vi "pmu_Build Time Quality Flag.vi"(0 "unlocked seconds":u32, 1 "synchronization error (s)":dbl=1e-07 format="%#_15f", 5 "locked?":bool, 7 "leap second pending":bool, 9 "leap second occurred":bool, 11 "leap second direction":bool) -> (4 "time quality flag":u8 format="%08b", 6 "PMU time quality":u8 format="%08b")   [LabVIEW 2013, in "NI_EP_PMU.lvlib"]
doc: "Outputs time quality flag bits, according to IEEE Std C37.118."
uses:
  <vilib>/addons/Electrical Power/PMU/NI_EP_PMU.lvlib
panel:
  # "100 ns"
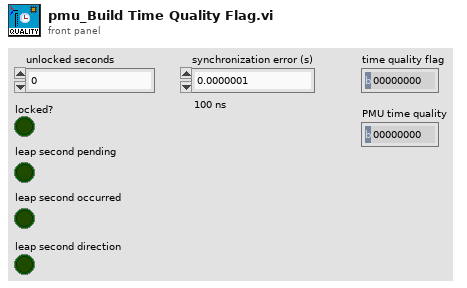
[diagram p1: front panel]
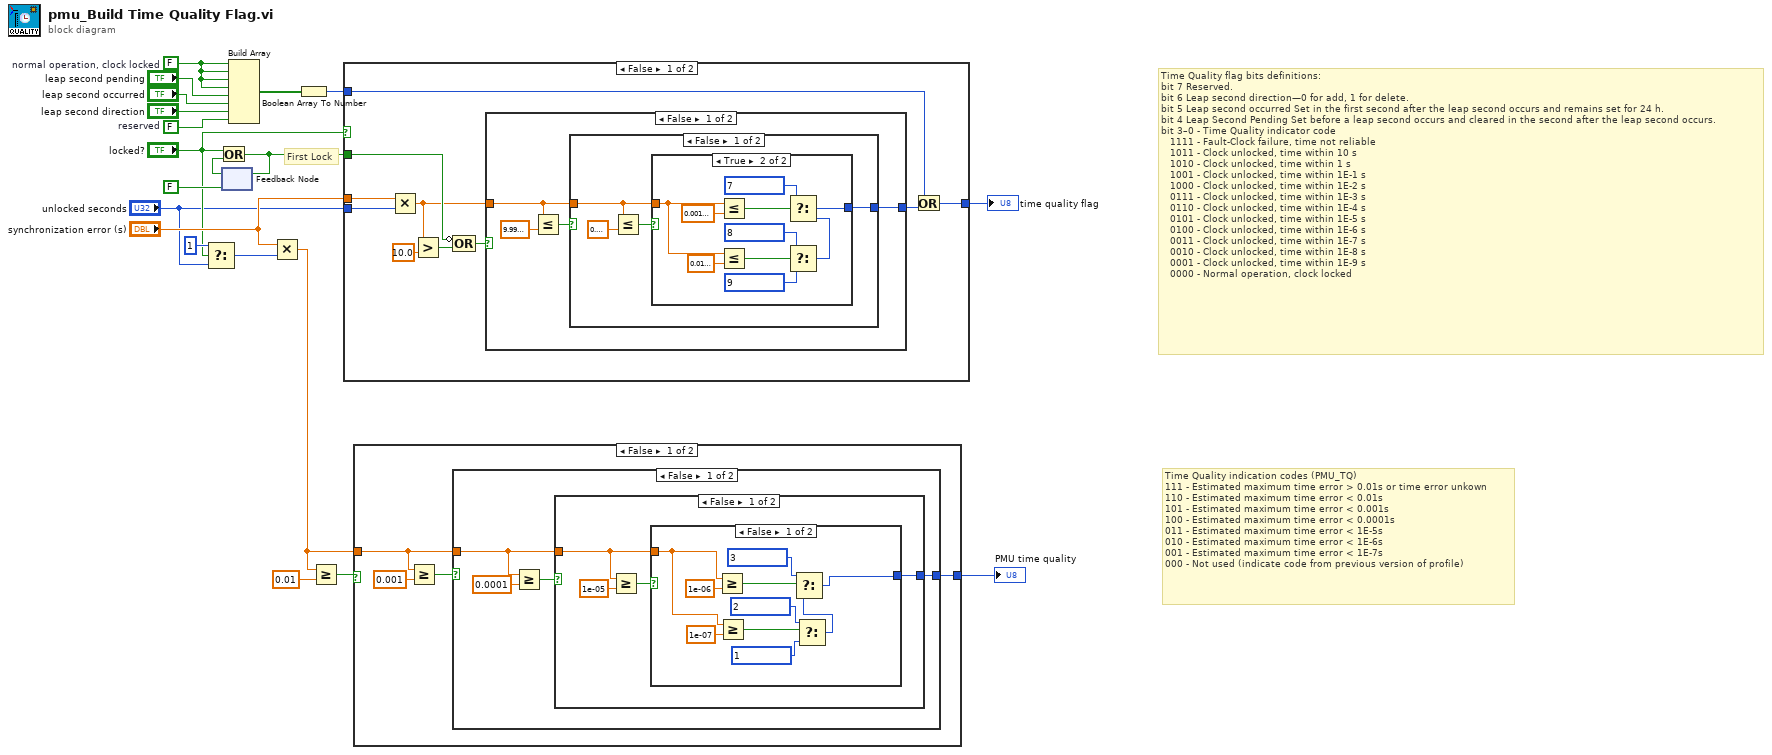
[diagram p0: block diagram]
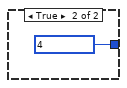
[diagram p2: hidden frame]
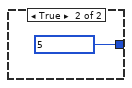
[diagram p3: hidden frame]
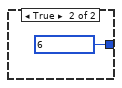
[diagram p4: hidden frame]
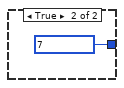
[diagram p5: hidden frame]
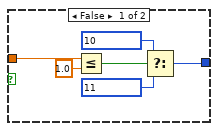
[diagram p6: hidden frame]
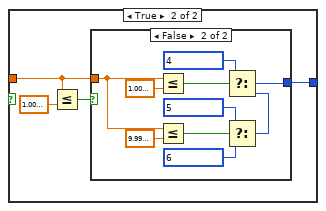
[diagram p7: hidden frame]
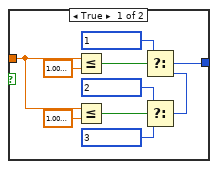
[diagram p8: hidden frame]
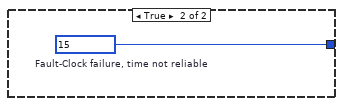
[diagram p9: hidden frame]
diagram:
  w11 = FALSE  # normal operation, clock locked
  w10 = FALSE  # reserved
  # "Time Quality indication codes (PMU_TQ)\n111 - Estimated maximum time error > 0.01s or time error unkown\n110 - Estimated maximum time error < 0.01s\n101 - Estimated maximum time error < 0.001s\n100 - Estimated maximum time error < 0.0001s\n011 - Estimated maximum time error < 1E-5s\n010 - Estimated maximum time error < 1E-6s\n001 - Estimated maximum time error < 1E-7s\n000 - Not used (indicate code from previous version of profile)"
  # "First Lock"
  # "Time Quality flag bits definitions:\nbit 7 Reserved.\nbit 6 Leap second direction—0 for add, 1 for delete.\nbit 5 Leap second occurred Set in the first second after the leap second occurs and remains set for 24 h.\nbit 4 Leap Second Pending Set before a leap second occurs and cleared in the second after the leap second occurs.\nbit 3–0 - Time Quality indicator code\n   1111 - Fault-Clock failure, time not reliable\n   1011 - Clock unlocked, time within 10 s\n   1010 - Clock unlocked, time within 1 s\n   1001 - Clock unlocked, time within 1E-1 s\n   1000 - Clock unlocked, time within 1E-2 s\n   0111 - Clock unlocked, time within 1E-3 s\n   0110 - Clock unlocked, time within 1E-4 s\n   0101 - Clock unlocked, time within 1E-5 s\n   0100 - Clock unlocked, time within 1E-6 s\n   0011 - Clock unlocked, time within 1E-7 s\n   0010 - Clock unlocked, time within 1E-8 s\n   0001 - Clock unlocked, time within 1E-9 s\n   0000 - Normal operation, clock locked"
  n1 = Select(t=u32 1, s="locked?", f="unlocked seconds") -> (s? t:f=w1:u32)
  n2 = feedback #1(FALSE) -> (w19:bool)
  n3 = Or(x="locked?", y=w19) -> (x .or. y?=w16:bool)
  n4 = feedback-in #1(w16) -> ()
  n5 = Build Array(w11, w11, w11, w11, "leap second pending", "leap second occurred", "leap second direction", w10) -> (w18:bool[])
  n6 = Multiply(x="synchronization error (s)", y=w1) -> (x*y=w5:dbl)
  n7 = Boolean Array To Number(Boolean array=w18) -> (number=w17:u8)
  n8 = Greater Or Equal?(x=w5, y=0.01) -> (x >= y?=w8:bool)
  n9 = case shown="False" "locked?" {
    tunnel: "unlocked seconds" -> [w22 _]
    tunnel: [w24 w80] -> w15
    tunnel: w17 -> [w25 w80]
    tunnel: w16 -> [w28 _]
    tunnel: "synchronization error (s)" -> [w21 _]
    frame False {
      n10 = Multiply(x=w21, y=w22) -> (x*y=w27:dbl)
      n11 = Greater?(x=w27, y=10.0) -> (0:w29:bool)
      n12 = Compound Arithmetic op=OR(invert w28, w29) -> (w26:bool)
      n13 = case shown="False" w26 {
        tunnel: [w31 w79] -> w23
        tunnel: w27 -> [w32 _]
        frame False {
          n14 = Less Or Equal?(x=w32, y=9.999999999976694e-05) -> (x <= y?=w33:bool)
          n15 = case shown="False" w33 {
            tunnel: w32 -> [w36 w56]
            tunnel: [w35 w55] -> w31
            frame False {
              n16 = Less Or Equal?(x=w36, y=0.10000000000000142) -> (x <= y?=w37:bool)
              n17 = case shown="True" w37 {
                tunnel: w36 -> [w43 w49]
                tunnel: [w39 w51] -> w35
                frame False {
                  n18 = Less Or Equal?(x=w43, y=1.0) -> (x <= y?=w42:bool)
                  n19 = Select(t=u8 10, s=w42, f=u8 11) -> (s? t:f=w39:u8)
                }
                frame True {
                  n20 = Less Or Equal?(x=w49, y=0.0010000000000012221) -> (x <= y?=w53:bool)
                  n21 = Less Or Equal?(x=w49, y=0.010000000000001563) -> (x <= y?=w48:bool)
                  n22 = Select(t=u8 8, s=w48, f=u8 9) -> (s? t:f=w45:u8)
                  n23 = Select(t=u8 7, s=w53, f=w45) -> (s? t:f=w51:u8)
                }
              }
            }
            frame True {
              n24 = Less Or Equal?(x=w56, y=1.0000000116860974e-07) -> (x <= y?=w57:bool)
              n25 = case shown="False" w57 {
                tunnel: w56 -> [w63 w73]
                tunnel: [w65 w75] -> w55
                frame True {
                  n26 = Less Or Equal?(x=w63, y=1.000000082740371e-09) -> (x <= y?=w67:bool)
                  n27 = Less Or Equal?(x=w63, y=1.000000082740371e-08) -> (x <= y?=w62:bool)
                  n28 = Select(t=u8 2, s=w62, f=u8 3) -> (s? t:f=w59:u8)
                  n29 = Select(t=u8 1, s=w67, f=w59) -> (s? t:f=w65:u8)
                }
                frame False {
                  n30 = Less Or Equal?(x=w73, y=1.0000000010279564e-06) -> (x <= y?=w77:bool)
                  n31 = Less Or Equal?(x=w73, y=9.999999999621423e-06) -> (x <= y?=w72:bool)
                  n32 = Select(t=u8 5, s=w72, f=u8 6) -> (s? t:f=w69:u8)
                  n33 = Select(t=u8 4, s=w77, f=w69) -> (s? t:f=w75:u8)
                }
              }
            }
          }
        }
        frame True {
          w79 = u8 15  # Fault-Clock failure, time not reliable
        }
      }
      n34 = Or(x=w25, y=w23) -> (x .or. y?=w24:u8)
    }
    frame True {
    }
  }
  "time quality flag" <- w15
  n35 = case shown="False" w8 {
    tunnel: [w82 u8 7] -> w6
    tunnel: w5 -> [w81 _]
    frame False {
      n36 = Greater Or Equal?(x=w81, y=0.001) -> (x >= y?=w83:bool)
      n37 = case shown="False" w83 {
        tunnel: [w86 u8 6] -> w82
        tunnel: w81 -> [w85 _]
        frame False {
          n38 = Greater Or Equal?(x=w85, y=0.0001) -> (x >= y?=w87:bool)
          n39 = case shown="False" w87 {
            tunnel: [w90 u8 5] -> w86
            tunnel: w85 -> [w89 _]
            frame False {
              n40 = Greater Or Equal?(x=w89, y=1e-05) -> (x >= y?=w91:bool)
              n41 = case shown="False" w91 {
                tunnel: [w93 u8 4] -> w90
                tunnel: w89 -> [w98 _]
                frame False {
                  n42 = Greater Or Equal?(x=w98, y=1e-06) -> (x >= y?=w101:bool)
                  n43 = Greater Or Equal?(x=w98, y=1e-07) -> (x >= y?=w97:bool)
                  n44 = Select(t=u8 2, s=w97, f=u8 1) -> (s? t:f=w94:u8)
                  n45 = Select(t=u8 3, s=w101, f=w94) -> (s? t:f=w93:u8)
                }
                frame True {
                }
              }
            }
            frame True {
            }
          }
        }
        frame True {
        }
      }
    }
    frame True {
    }
  }
  "PMU time quality" <- w6
